vi "LookupNodeByName.vi"(8 "error in (no error)":errorcluster, 10 "Python Node Name":string, 11 "Server in":refnum<class "Server.lvclass">) -> (0 "error out":errorcluster, 1 "Found?":bool, 2 "PYTHON Node":T1, 3 "Server out":refnum<class "Server.lvclass">)   [LabVIEW 2013, in "JKI_Python_Bridge_for_LV.lvlib" / "Server.lvclass"]
uses:
  Server.lvclass
  Type Definitions/Python Node.ctl
  CallHandler/CallHandler.lvclass
  Call/Call.lvclass
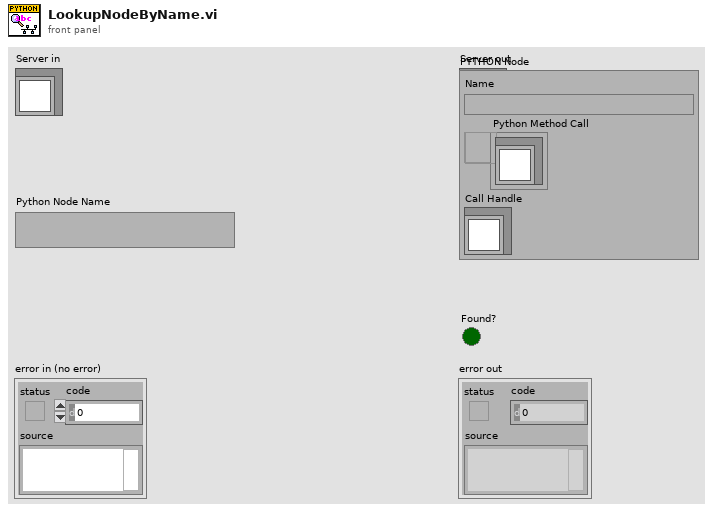
[diagram p1: front panel]
types:
  T1 = typedef "JKI_Python_Bridge_for_LV.lvlib/Server.lvclass/Python Node.ctl" = cluster{"Name":string, "Python Method Call":refnum<user-event>, "Call Handle":refnum<class "CallHandler.lvclass">}
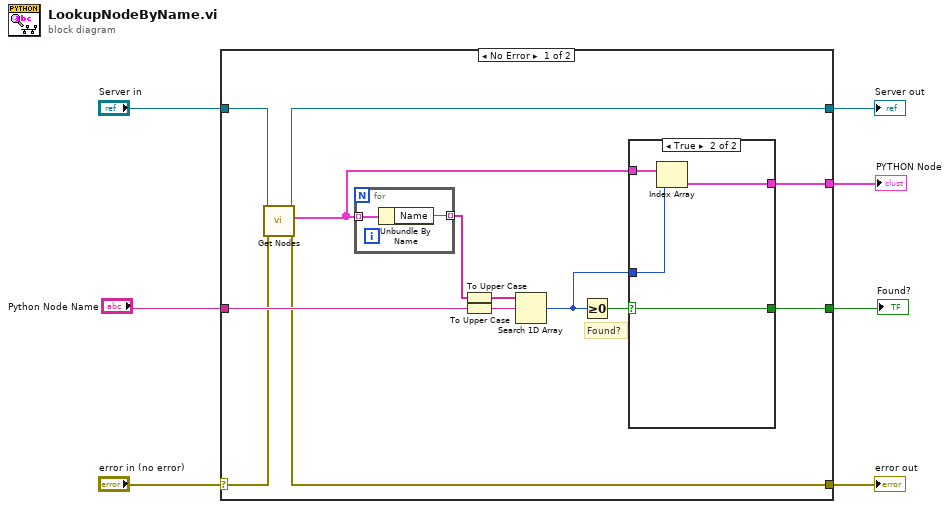
[diagram p0: block diagram]
diagram:
  n1 = case shown="No Error" "error in (no error)" {
    selector: "error in (no error)" -> [w12 w29]
    tunnel: [w11 w29] -> w6
    tunnel: [w9 w28] -> w4
    tunnel: "Server in" -> [w10 w28]
    tunnel: "Python Node Name" -> [w14 _]
    tunnel: [w13 _] -> w2
    tunnel: [w8 _] -> w1
    frame No Error {
      # "Found?"
      n2 = call "Get Nodes.vi"("error in (no error)"=w12, "JKI_Python_Server in"=w10) -> ("error out"=w11:errorcluster, "Nodes"=w15:T1[], "JKI_Python_Server out"=w9:refnum<class "Server.lvclass">)  [unwired: 7 in]
      n3 = for {
        tunnel: w15 -> [w27] mode=indexing
        tunnel: [w26] -> w18 mode=indexing
        n4 = Unbundle By Name(w27) -> ("Name"=w26:string)
      }
      n5 = To Upper Case(1:w18) -> (0:w17:string[])
      n6 = To Upper Case(1:w14) -> (0:w16:string)
      n7 = Search 1D Array(1D array=w17, element=w16) -> (index of element=w19:i32)  [unwired: 1 in]
      n8 = Greater Or Equal To 0?(x=w19) -> (x >= 0?=w20:bool)
      n9 = case shown="True" w20 {
        selector: w20 -> [w21 w22]
        tunnel: w15 -> [_ w25]
        tunnel: w19 -> [_ w24]
        tunnel: [_ w23] -> w13
        tunnel: [w21 w22] -> w8
        frame False {
        }
        frame True {
          n10 = Index Array(array=w25, index=w24) -> (element=w23:T1)
        }
      }
    }
    frame Error {
    }
  }
  "error out" <- w6
  "Server out" <- w4
  "PYTHON Node" <- w2
  "Found?" <- w1
